vi "RSNRPZ Get Statistics Scale Width.vi"(8 "error in (no error)":errorcluster, 10 "Channel (1)":i32=1, 11 "VISA session":refnum<visa-resource-name> caption="VISA resource name") -> (0 "error out":errorcluster, 2 "Width":dbl format="%^.3e", 3 "dup VISA session":refnum<visa-resource-name> caption="VISA resource name")   [LabVIEW 2010]
doc: "This VI queries the greatest attainable level resolution. For the R&S NRP-Z81 power sensor, this value is fixed at 0.006 dB per pixel. If this value is exceeded, a \"Settings conflict\" message is output. The reason for the conflict may be that the number of pixels that has been selected is too great or that the width chosen for the level range is too small (rsnrpz_stat_setScalePoints and rsnrpz_stat_setScaleRange VIs).\n\nRemote-control command(s):\nSENSe:STATistics:SCALE:X:MPWidth?"
uses:
  rsnrpz_32.dll
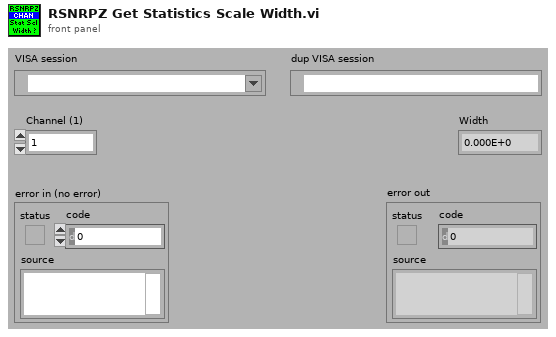
[diagram p1: front panel]
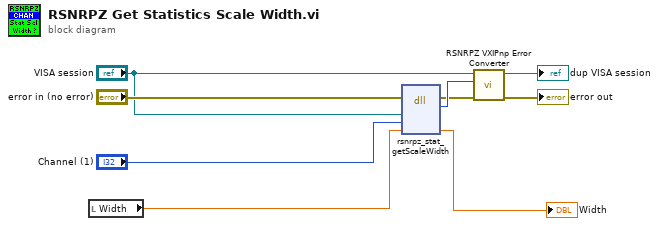
[diagram p0: block diagram]
diagram:
  n1 = local read "Width"() -> (w7:dbl)
  n2 = dll-call lib="rsnrpz_32.dll" fn="rsnrpz_stat_getScaleWidth"(error in="error in (no error)", "Instrument Handle"="VISA session", "Channel"="Channel (1)", "Width"=w7) -> (error out=w5:errorcluster, "Status"=w9:i32, "Width"=→"Width":dbl)  [unwired: 4 in, 1 out]
  n3 = call <instrlib>:"RSNRPZ VXIPnp Error Converter.vi"("error in"=w5, "VXIPnp error code"=w9, "VISA session"="VISA session") -> ("error out"=→"error out":errorcluster, "dup VISA session"=→"dup VISA session":refnum<visa-resource-name>)  [unwired: 7 in]
